vi "FormInfo.vi"   [LabVIEW 2012]
panel:
  # "广东和氏自动化技术股份有限公司"
  # "GUANGDONG HESH AUTOMATION TECHNOLOGY CO.,LTD."
  # "广东和氏自动化技术股份有限公司位于中国南方美丽的海滨城市珠海。和氏公司是于2003年成立的技术型生产企业。公司是以“改善客户的效率、安全和环境”为宗旨，从事非标自动化设备、精密器材、模具、机械零件的开发，设计、制造的专业化公司。\n和氏公司凭借科学的经营理念，执着的创新追求，务实的工作作风使产品广泛用于汽车、空调、制冷压缩机、电子、家用电器、机械制造、金属材料加工等行业。\n和氏秉承以人为本的原则，聚集了一批产品开发设计、制造加工、安装调试、售后服务的专业人才，有能力为客户提供独特的产品和技术服务。 \n和氏期待与广大合作伙伴共同发展与成功！"
  # "合肥和氏自动化技术有限公司是珠海和氏自动化设备有限公司全资公司。合肥和氏秉承着珠海和氏的方针和宗旨，致力于先进自动化装备的研发、制造和服务，公司拥有高素质的研发队伍、先进的制造设备、以及高品质的制造水平，注重团队精神的建设。\n公司地址: 安徽省合肥市高新区科学大道与红枫路交口（中瑞大厦A座1306室）\n联系方式:0551-65302130   qq:896720082"
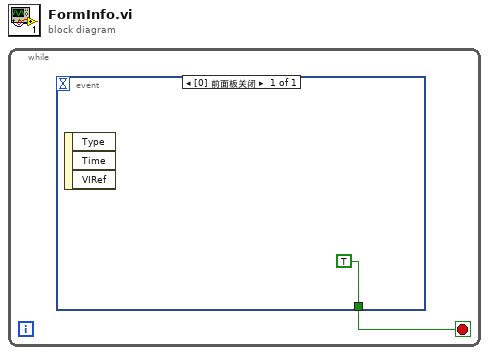
[diagram p0: block diagram]
diagram:
  n1 = while {
    stop <- w1 stop-if-true
    n2 = event shown="[0] 前面板关闭" {
      selector: _ -> [_]
      dyn-events: _ -> [_]
      timeout: _ -> [_]
      tunnel: [TRUE] -> w1
      event Panel Close {
        n3 = event-data() -> ()  [unwired: 1 in, 3 out]
      }
    }
  }
